vi "Grave Left Cell.vi"(8 "Error In":errorcluster, 10 "Bookmark ID":u32, 11 "VI Info":T1) -> (0 "Error Out":errorcluster, 1 "Bold?":bool, 2 "Color":u32(colorbox)=40705, 3 "Text":string)   [LabVIEW 2017, in "Bookmark Manager.lvlib"]
doc: "Gets the state name of the grave. If the Spirit frame is enabled, then the name is \"Spirit\". If the Corpse frame is enabled, then the name is \"Zombie\".\n\nThe Diagram Disable Structure cannot be obtained its label. The owning object of the label is the block diagram, not the Diagram Disable Structure that is attached to it. This means that all of the Diagram Disable structures in a VI must be searched by their label's UIDs to find the Diagram Disable Structure and determine its state."
uses:
  Bookmark Manager.lvlib
  Controls/VI Information.ctl
  Controls/Application Information.ctl
  Controls/Grave States.ctl
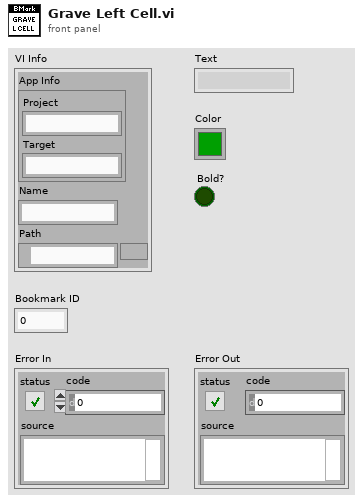
[diagram p1: front panel]
types:
  T1 = typedef "Bookmark Manager.lvlib/VI Information.ctl" = cluster{"App Info":T2, "Name":string, "Path":path}
  T2 = typedef "Bookmark Manager.lvlib/Application Information.ctl" = cluster{"Project":string, "Target":string}
  T3 = typedef "Bookmark Manager.lvlib/Grave States.ctl" = enum16{"Spirit", "Zombie"}
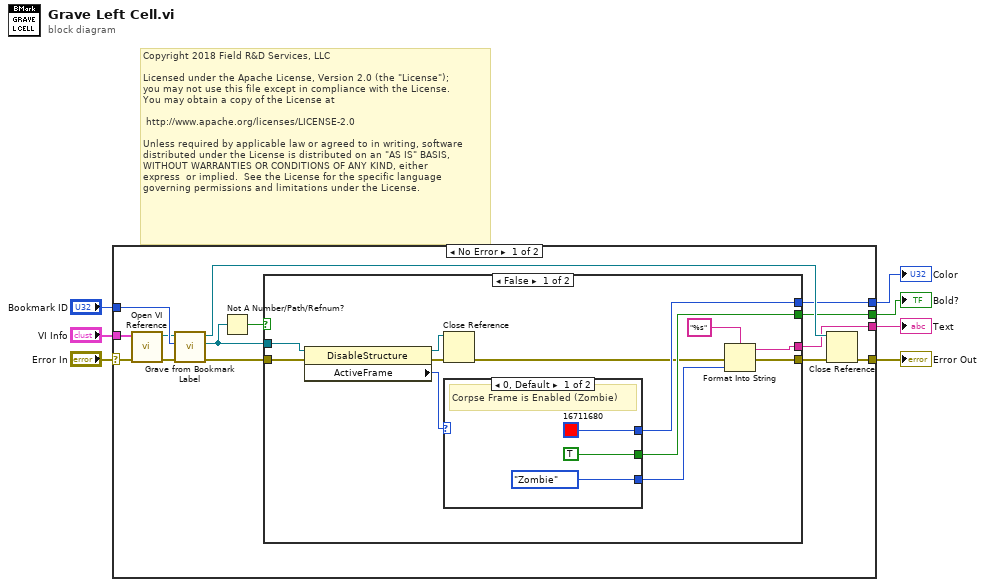
[diagram p0: block diagram]
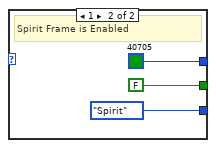
[diagram p2: hidden frame]
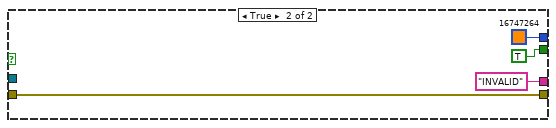
[diagram p3: hidden frame]
diagram:
  # "Copyright 2018 Field R&D Services, LLC\n\nLicensed under the Apache License, Version 2.0 (the \"License\");\nyou may not use this file except in compliance with the License.\nYou may obtain a copy of the License at\n\n\thttp://www.apache.org/licenses/LICENSE-2.0\n\nUnless required by applicable law or agreed to in writing, software\ndistributed under the License is distributed on an \"AS IS\" BASIS,\nWITHOUT WARRANTIES OR CONDITIONS OF ANY KIND, either \nexpress  or implied.  See the License for the specific language \ngoverning permissions and limitations under the License."
  n1 = case shown="No Error" "Error In" {
    selector: "Error In" -> [w17 w44]
    tunnel: [w13 w44] -> w7
    tunnel: [w19 _] -> w6
    tunnel: "VI Info" -> [w10 _]
    tunnel: "Bookmark ID" -> [w18 _]
    tunnel: [w16 _] -> w2
    tunnel: [w15 _] -> w1
    frame No Error {
      n2 = call "Open VI Reference.vi"("Error In"=w17, "VI Info"=w10) -> ("Error Out"=w9:errorcluster, "VI"=w8:refnum<vi>)  [unwired: 8 in]
      n3 = call "Grave from Bookmark Label.vi"("Error In"=w9, "Bookmark ID"=w18, "VI In"=w8) -> ("Error Out"=w21:errorcluster, "Grave"=w12:refnum<vi>, "VI Out"=w20:refnum<vi>)  [unwired: 6 in]
      n4 = Not A Number/Path/Refnum?(number/path/refnum=w12) -> (NaN/Path/Refnum?=w11:bool)
      n5 = case shown="False" w11 {
        tunnel: w21 -> [w31 w41]
        tunnel: [w28 "INVALID"] -> w19
        tunnel: [w26 u32 16747264] -> w16
        tunnel: [w25 TRUE] -> w15
        tunnel: [w23 w41] -> w14
        tunnel: w12 -> [w22 _]
        frame False {
          n6 = property class="DisableStructure"(reference=w22, error in=w31) -> (reference out=w27:refnum<vi>, error out=w32:errorcluster, "ActiveFrame"=w33:i16)
          n7 = Close Reference(reference=w27, error in (no error)=w32) -> (error out=w24:errorcluster)
          n8 = case shown="0, Default" w33 {
            tunnel: [Grave_States."Zombie" ("Grave States") Grave_States."Spirit" ("Grave States")] -> w30
            tunnel: [u32 16711680 u32 40705] -> w26
            tunnel: [TRUE FALSE] -> w25
            frame 0, Default {
              # "Corpse Frame is Enabled (Zombie)"
            }
            frame 1 {
              # "Spirit Frame is Enabled"
            }
          }
          n9 = Format Into String(format string="%s", error in=w24, w30) -> (resulting string=w28:string, error out=w23:errorcluster)  [unwired: 1 in]
        }
        frame True {
        }
      }
      n10 = Close Reference(reference=w20, error in (no error)=w14) -> (error out=w13:errorcluster)
    }
    frame Error {
    }
  }
  "Error Out" <- w7
  "Text" <- w6
  "Color" <- w2
  "Bold?" <- w1
